vi "Name Label Size Read.vi"(8 "error in (no error)":errorcluster, 11 "3D Plot.lvclass in":refnum<class "3D Plot.lvclass">) -> (0 "error out":errorcluster, 1 "Caption Font Size":u16, 3 "3D Plot.lvclass out":refnum<class "3D Plot.lvclass">)   [LabVIEW 2020, in "3D Plot.lvclass"]
uses:
  3D Plot.lvclass
  3D Plot.lvclass/3D Plot.ctl
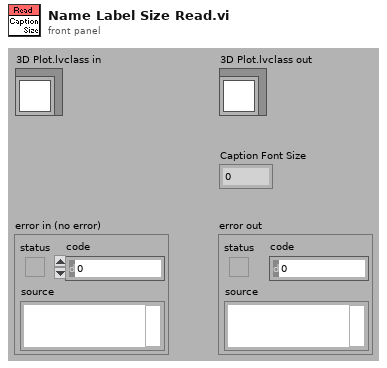
[diagram p1: front panel]
types:
  T1 = cluster{"Caption Size X":u16, "Caption Size Y":u16, "Caption Size Z":u16}
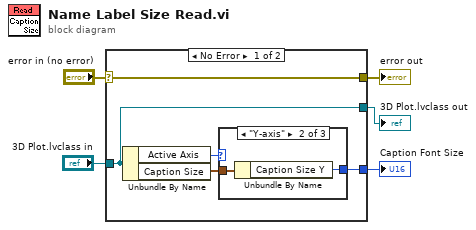
[diagram p0: block diagram]
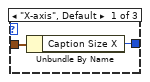
[diagram p2: hidden frame]
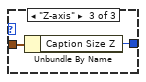
[diagram p3: hidden frame]
diagram:
  n1 = case shown="No Error" "error in (no error)" {
    selector: "error in (no error)" -> [w6 w17]
    tunnel: [w10 _] -> w5
    tunnel: "3D Plot.lvclass in" -> [w7 w18]
    tunnel: [w7 w18] -> w3
    tunnel: [w6 w17] -> w1
    frame No Error {
      n2 = Unbundle By Name(w7) -> ("Active Axis"=w8:enum16{"X-axis", "Y-axis", "Z-axis"}, "Caption Size"=w9:T1)
      n3 = case shown="\"Y-axis\"" w8 {
        tunnel: w9 -> [w11 w14 w16]
        tunnel: [w12 w13 w15] -> w10
        frame "X-axis", Default {
          n4 = Unbundle By Name(w11) -> ("Caption Size X"=w12:u16)
        }
        frame "Y-axis" {
          n5 = Unbundle By Name(w14) -> ("Caption Size Y"=w13:u16)
        }
        frame "Z-axis" {
          n6 = Unbundle By Name(w16) -> ("Caption Size Z"=w15:u16)
        }
      }
    }
    frame Error {
    }
  }
  "error out" <- w1
  "Caption Font Size" <- w5
  "3D Plot.lvclass out" <- w3
